vi "FPGA-Balanced_IO.vi"() -> ()   [LabVIEW 2014]
uses:
  <vilib>/eio/EIONode/EIONode.xnode
  <vilib>/Platform/TimedLoop/XDataNode/wakeup.ctl
  <vilib>/Platform/TimedLoop/XDataNode/XDNodeRunTimeDep.lvlib
  <vilib>/Platform/TimedLoop/XDataNode/nitl_modes.ctl
  <vilib>/Platform/TimedLoop/XDataNode/timing_clust.ctl
  <vilib>/Platform/TimedLoop/XDataNode/XDataNode.xnode
  <vilib>/rvi/DataTransferAndStorage/Container/XNode/niFpgaContainer.xnode
  <vilib>/rvi/eio/common/nirviEmuTemplateMethod_errors.vi
  <vilib>/rvi/interface/RandomDataEmulation/nirviRandomDataFpgaReadWriteTemplate.vi
panel:
  out "AO: Actual Loop Rate(ticks)":u32
  in  "AO 0":i16
  in  "AO 1":i16
  in  "AO 2":i16
  in  "AO 3":i16
  in  "AO 4":i16
  in  "AO 5":i16
  in  "AO 6":i16
  in  "AO 7":i16
  in  "AO Loop Timer(Ticks)":u32
  out "AO Buffer Underflow?":bool
  in  "AO Buffer Enable":u8 format="%08b"
  in  "AO Enable":bool
  in  "AI Channel Enable":u8
  out "AI: Actual Loop Rate (ticks)":u32
  in  "AI Enable":bool
  out "AI Counter":u32
  out "AI Buffer Overflow?":bool
  in  "AI Loop Timer(Ticks)":u32
  # "Analog Output"
  # "Analog Input"
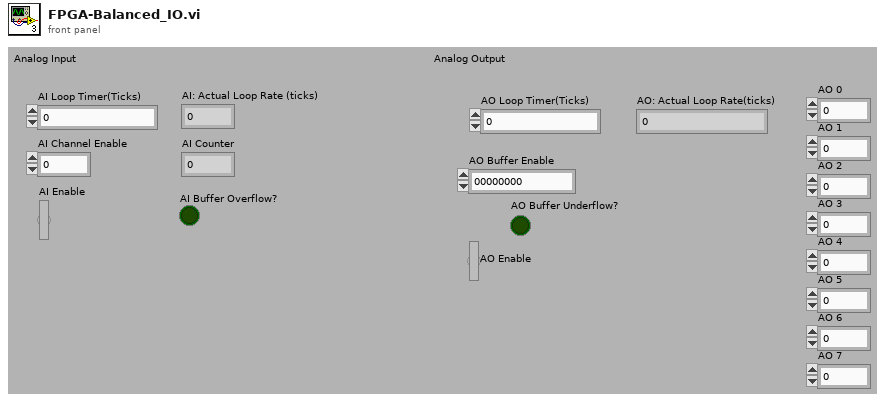
[diagram p1: front panel]
types:
  T1 = typedef "XDNodeRunTimeDep.lvlib/timing_clust.ctl" = cluster{"Expected End [f-1]":u64, "Actual End [f-1]":u64, "Finished Late? [f-1]":bool, "Expected End [i-1]":u64, "Actual End [i-1]":u64, "Finished Late? [i-1]":bool, "Expected Start [i]":u64, "Actual Start [i]":u64, "Expected Start [f]":u64, "Actual Start [f]":u64, "Source Name":string, "Structure Name":string, "Period":i64, "Deadline":i64, "Offset":i64, "Start":i64, "Priority":i32, "Timeout":i32, "Mode":T2, "Wakeup Reason":T3, "Error":errorcluster, "Source Type":string, "Secondary Source Type":string, "Global End Time":u64, "Global Start Time":u64, "Frame Duration":u64, "Iteration Duration":u64, "Assigned CPU":i32, "I/O Scan Engine Mode":u32}
  T2 = typedef "XDNodeRunTimeDep.lvlib/nitl_modes.ctl" = enum32{"No Change", "Process missed periods, maintain original phase", "Discard missed periods, maintain original phase", "Process missed periods, ignore original phase", "Discard missed periods, ignore original phase"}
  T3 = typedef "XDNodeRunTimeDep.lvlib/wakeup.ctl" = enum32{"Normal", "Aborted", "Asynchronous wakeup", "Timing source error", "Timed loop error", "Timeout"}
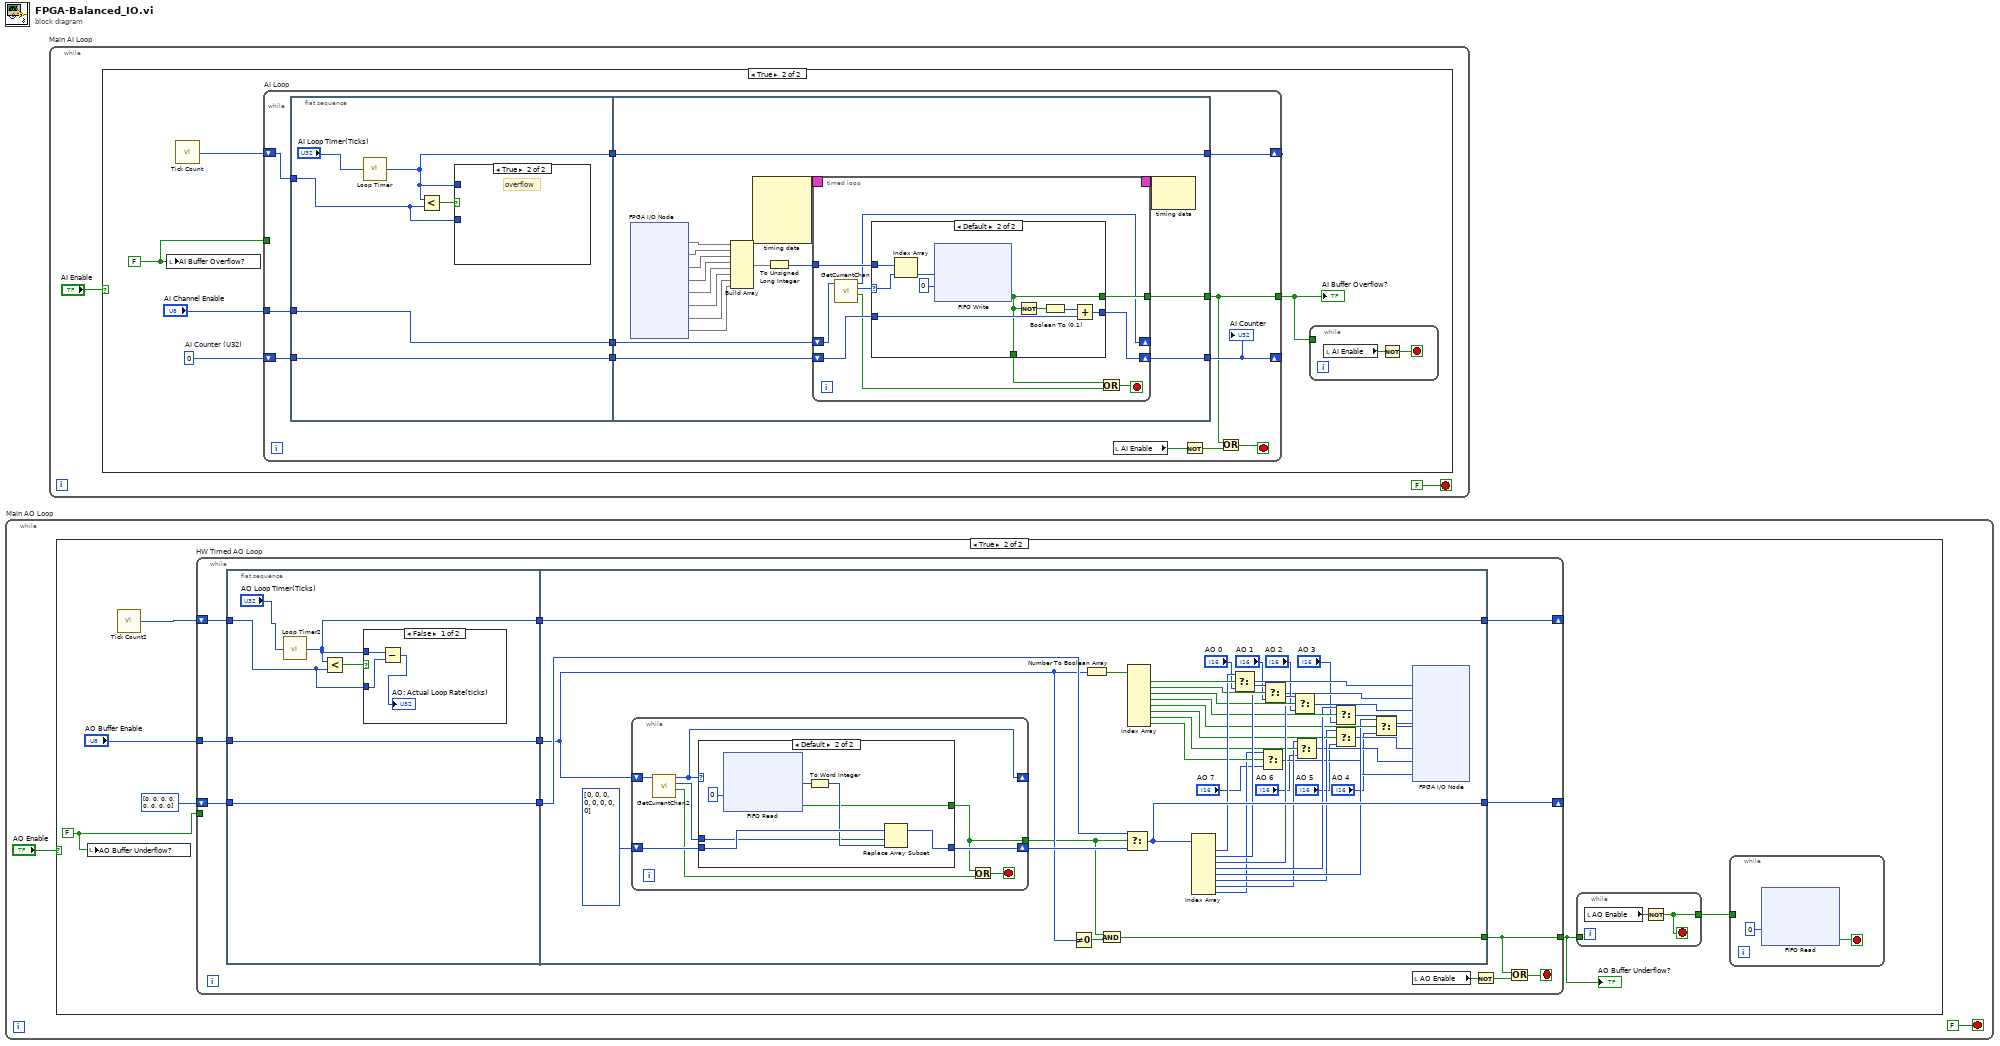
[diagram p0: block diagram]
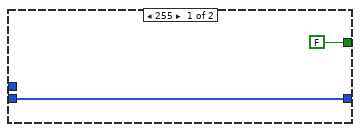
[diagram p4: hidden frame]
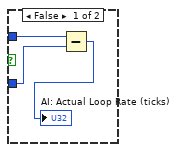
[diagram p6: hidden frame]
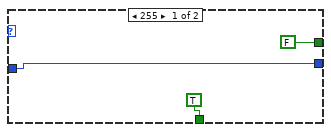
[diagram p7: hidden frame]
diagram:
  n1 = while "Main AO Loop" {
    stop <- FALSE stop-if-true
    n2 = case shown="True" "AO Enable" {
      frame False {
      }
      frame True {
        w8 = FALSE ("AO Buffer Underflow?")
        n3 = local write "AO Buffer Underflow?"(w8) -> ()
        n4 = call "Tick Count2"() -> ("Tick Count(Ticks)"=w3:u32)
        n5 = while "HW Timed AO Loop" {
          tunnel: [w23] -> w5
          tunnel: w8 -> [_]
          tunnel: "AO Buffer Enable" -> [w20]
          shift-right: [w18] -> _
          shift-left: i16[] [0, 0, 0, 0, 0, 0, 0, 0] -> [w17]
          shift-right: [w14] -> _
          shift-left: w3 -> [w13]
          stop <- w24 stop-if-true
          n6 = flat-sequence {
            tunnel: w20 -> [w30]
            tunnel: [w30] -> w19
            tunnel: w17 -> [w29]
            tunnel: [w29] -> w16
            tunnel: [w25] -> w15
            tunnel: w13 -> [w27]
            tunnel: [w34] -> w23
            tunnel: w19 -> [w37]
            tunnel: [w71] -> w18
            tunnel: w16 -> [w70]
            tunnel: w15 -> [w38]
            tunnel: [w38] -> w14
            frame #0 {
              n7 = call "Loop Timer2"("Count(Ticks)"="AO Loop Timer(Ticks)") -> ("Tick Count(Ticks)"=w25:u32)
              n8 = Less?(x=w25, y=w27) -> (x < y?=w28:bool)
              n9 = case shown="False" w28 {
                tunnel: w25 -> [w33 _]
                tunnel: w27 -> [w32 _]
                frame False {
                  n10 = Subtract(x=w33, y=w32) -> (x-y=→"AO: Actual Loop Rate(ticks)":u32)
                }
                frame True {
                  # "overflow"
                }
              }
            }
            frame #1 {
              n11 = while {
                shift-right: [w82] -> w72
                shift-left: i16[] [0, 0, 0, 0, 0, 0, 0, 0] -> [w83]
                tunnel: [w76] -> w35
                shift-right: [w80] -> _
                shift-left: w37 -> [w81]
                stop <- w77 stop-if-true
                n12 = call "GetCurrentChan2.vi"("AI Select In"=w81) -> ("Stop Loop"=w78:bool, "Current Channel"=w79:u8, "AI Select Out"=w80:u8)  [unwired: 8 in]
                n13 = case shown="Default" w80 {
                  tunnel: w83 -> [w84 w90]
                  tunnel: [w84 w89] -> w82
                  tunnel: [FALSE ("Empty") w86] -> w76
                  tunnel: w79 -> [_ w87]
                  frame 255 {
                  }
                  frame Default {
                    n14 = xnode ("FIFO Read")("Timeout"=0) -> ("Element"=w91:u32, "Timed Out?"=w86:bool)  [unwired: 1 in, 1 out]
                    n15 = To Word Integer(number=w91) -> (16bit integer=w88:i16)
                    n16 = Replace Array Subset(array=w90, new element=w88, index=w87) -> (w89:i16[])
                  }
                }
                n17 = Or(x=w76, y=w78) -> (x .or. y?=w77:bool)
              }
              n18 = Not Equal To 0?(x=w37) -> (x != 0?=w36:bool)
              n19 = Number To Boolean Array(number=w37) -> (Boolean array=w74:bool[])
              n20 = And(x=w35, y=w36) -> (x .and. y?=w34:bool)
              n21 = Select(t=w70, s=w35, f=w72) -> (s? t:f=w71:i16[])
              n22 = Index Array(array=w74) -> (element #1=w73:bool, element #2=w67:bool, element #3=w65:bool, element #4=w58:bool, element #5=w54:bool, element #6=w53:bool, element #7=w52:bool, element #8=w51:bool)  [unwired: 8 in]
              n23 = Index Array(array=w71) -> (element #1=w69:i16, element #2=w66:i16, element #3=w64:i16, element #4=w57:i16, element #5=w50:i16, element #6=w49:i16, element #7=w48:i16, element #8=w47:i16)  [unwired: 8 in]
              n24 = Select(t=w69, s=w73, f="AO 0") -> (s? t:f=w68:i16)
              n25 = Select(t=w47, s=w51, f="AO 7") -> (s? t:f=w43:i16)
              n26 = Select(t=w66, s=w67, f="AO 1") -> (s? t:f=w60:i16)
              n27 = Select(t=w64, s=w65, f="AO 2") -> (s? t:f=w59:i16)
              n28 = Select(t=w48, s=w52, f="AO 6") -> (s? t:f=w44:i16)
              n29 = Select(t=w57, s=w58, f="AO 3") -> (s? t:f=w55:i16)
              n30 = Select(t=w49, s=w53, f="AO 5") -> (s? t:f=w45:i16)
              n31 = Select(t=w50, s=w54, f="AO 4") -> (s? t:f=w46:i16)
              n32 = xnode "FPGA I/O Node"("AO0"=w68, "AO1"=w60, "AO2"=w59, "AO3"=w55, "AO4"=w46, "AO5"=w45, "AO6"=w44, "AO7"=w43) -> ()  [unwired: 8 in, 8 out]
            }
          }
          n33 = local read "AO Enable"() -> (w22:bool)
          n34 = Not(x=w22) -> (.not. x?=w21:bool)
          n35 = Or(x=w23, y=w21) -> (x .or. y?=w24:bool)
        }
        "AO Buffer Underflow?" <- w5
        n36 = while {
          tunnel: w5 -> [_]
          tunnel: [w11] -> w4
          stop <- w11 stop-if-true
          n37 = local read "AO Enable"() -> (w12:bool)
          n38 = Not(x=w12) -> (.not. x?=w11:bool)
        }
        n39 = while {
          tunnel: w4 -> [_]
          stop <- w9 stop-if-true
          n40 = xnode ("FIFO Read")("Timeout"=0) -> ("Timed Out?"=w9:bool)  [unwired: 1 in, 2 out]
        }
      }
    }
  }
  n41 = while "Main AI Loop" {
    stop <- FALSE stop-if-true
    n42 = case shown="True" "AI Enable" {
      frame False {
      }
      frame True {
        w98 = FALSE ("AI Buffer Overflow?")
        w99 = u32 0  # AI Counter (U32)
        n43 = local write "AI Buffer Overflow?"(w98) -> ()
        n44 = call "Tick Count"() -> ("Tick Count(Ticks)"=w95:u32)
        n45 = while "AI Loop" {
          shift-right: [w111] -> _
          shift-left: w99 -> [w112]
          tunnel: [w106] -> w96
          tunnel: w98 -> [_]
          shift-right: [w108] -> _
          shift-left: w95 -> [w107]
          tunnel: "AI Channel Enable" -> [w105]
          stop <- w110 stop-if-true
          n46 = flat-sequence {
            tunnel: [w119] -> w113
            tunnel: w112 -> [w119]
            tunnel: [w114] -> w109
            tunnel: w107 -> [w116]
            tunnel: w105 -> [w118]
            tunnel: [w118] -> w104
            tunnel: w113 -> [w127]
            tunnel: [w126] -> w111
            tunnel: w109 -> [w125]
            tunnel: [w125] -> w108
            tunnel: [w124] -> w106
            tunnel: w104 -> [w123]
            frame #0 {
              n47 = call "Loop Timer"("Count(Ticks)"="AI Loop Timer(Ticks)") -> ("Tick Count(Ticks)"=w114:u32)
              n48 = Less?(x=w114, y=w116) -> (x < y?=w117:bool)
              n49 = case shown="True" w117 {
                tunnel: w114 -> [w122 _]
                tunnel: w116 -> [w121 _]
                frame False {
                  n50 = Subtract(x=w122, y=w121) -> (x-y=→"AI: Actual Loop Rate (ticks)":u32)
                }
                frame True {
                  # "overflow"
                }
              }
            }
            frame #1 {
              n51 = xnode "FPGA I/O Node"() -> ("AI0"=w136, "AI1"=w139, "AI2"=w138, "AI3"=w137, "AI4"=w135, "AI5"=w134, "AI6"=w133, "AI7"=w132)  [unwired: 8 in, 8 out]
              n52 = Build Array(w136, w139, w138, w137, w135, w134, w133, w132) -> (w131:void[])
              n53 = node-c288() -> (w130:T1)  [unwired: 4 in]
              n54 = To Unsigned Long Integer(number=w131) -> (unsigned 32bit integer=w128:u32[])
              n55 = timed-loop {
                timing: w130 -> [_]
                timing-out: [_] -> w129
                tunnel: w128 -> [w149]
                shift-right: [w147] -> w126
                shift-left: w127 -> [w148]
                tunnel: [w146] -> w124
                shift-right: [w143] -> _
                shift-left: w123 -> [w145]
                stop <- w141 stop-if-true
                n56 = call "GetCurrentChan.vi"("AI Select In"=w145) -> ("Stop Loop"=w142:bool, "Current Channel"=w144:u8, "AI Select Out"=w143:u8)  [unwired: 8 in]
                n57 = case shown="Default" w144 {
                  selector: w144 -> [_ w155]
                  tunnel: w149 -> [_ w156]
                  tunnel: w148 -> [w150 w159]
                  tunnel: [w150 w158] -> w147
                  tunnel: [FALSE ("Full") w153] -> w146
                  tunnel: [TRUE ("Full") w153] -> w140
                  frame 255 {
                  }
                  frame Default {
                    n58 = Index Array(array=w156, index=w155) -> (element=w154:u32)
                    n59 = xnode ("FIFO Write")("Element"=w154, "Timeout"=0) -> ("Timed Out?"=w153:bool)  [unwired: 1 in, 1 out]
                    n60 = Not(x=w153) -> (.not. x?=w161:bool)
                    n61 = Boolean To (0,1)(Boolean=w161) -> (0, 1=w160:i16)
                    n62 = Add(x=w160, y=w159) -> (x+y=w158:u32)
                  }
                }
                n63 = Or(x=w140, y=w142) -> (x .or. y?=w141:bool)
              }
              n64 = node-c288(w129) -> ()  [unwired: 1 out]
            }
          }
          n65 = local read "AI Enable"() -> (w103:bool)
          n66 = Not(x=w103) -> (.not. x?=w102:bool)
          n67 = Or(x=w106, y=w102) -> (x .or. y?=w110:bool)
          "AI Counter" <- w111
        }
        "AI Buffer Overflow?" <- w96
        n68 = while {
          tunnel: w96 -> [_]
          stop <- w100 stop-if-true
          n69 = local read "AI Enable"() -> (w101:bool)
          n70 = Not(x=w101) -> (.not. x?=w100:bool)
        }
      }
    }
  }
